vi "carwash_test.vi"() -> ()   [LabVIEW 2017]
panel:
  in  "Wash Selec.":enum16{"Initialize", "Deluxe", "Economy"}(ring)
  out "Vehicle Out of Position":bool
  out "Air Dry":bool
  out "Clear Water Rinse":bool
  out "Main High Press. Wash":bool
  out "Soap Application":bool
  out "Under body Wash":bool
  in  "?":bool
  in  "?":bool
  in  "?":bool
  in  "stop":bool
  # "Car Wash Indicators"
  # "Underbody wash\nposition \nSwitch"
  # "Main Wash \nPosition \nSwitch"
  # "Air Dry\nPosition\nSwitch"
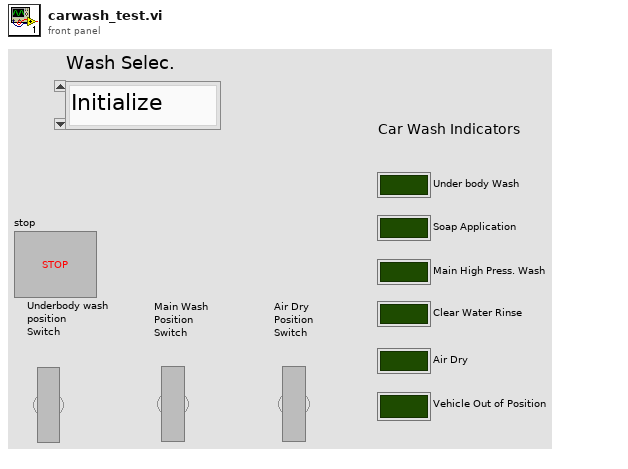
[diagram p1: front panel]
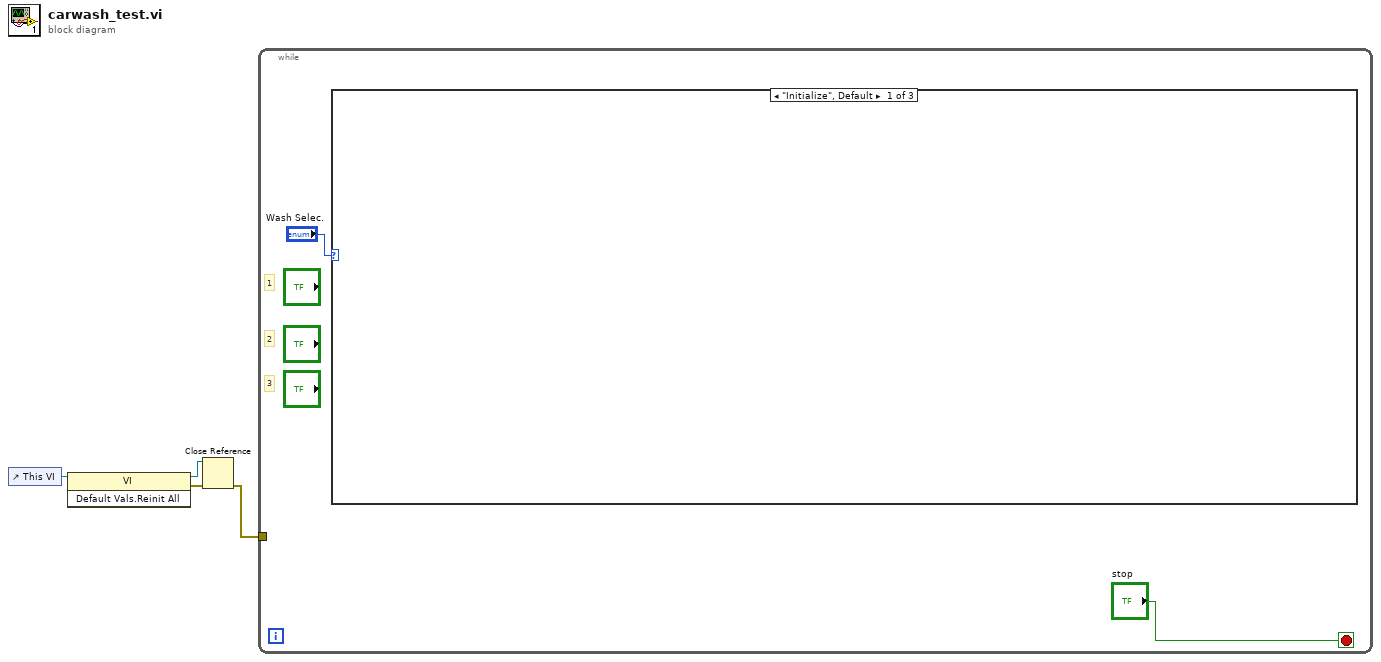
[diagram p0: block diagram]
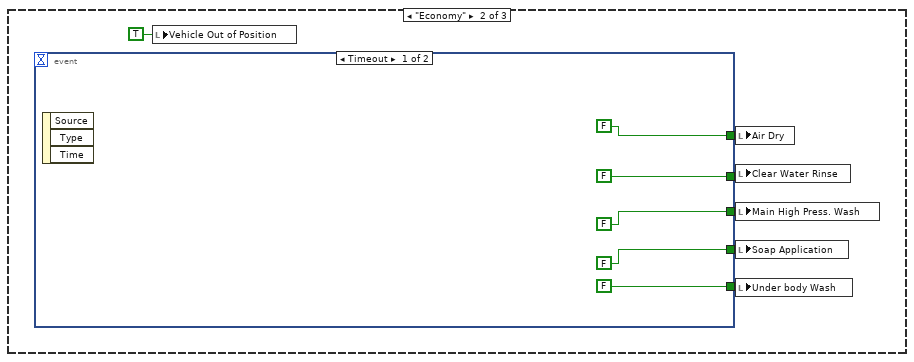
[diagram p2: hidden frame]
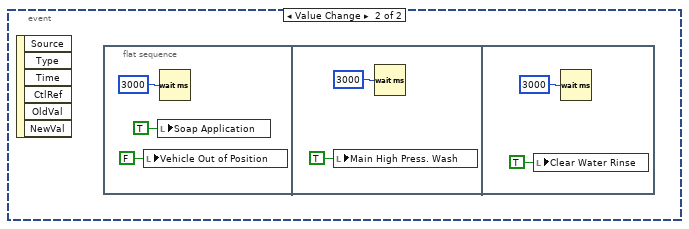
[diagram p3: hidden frame]
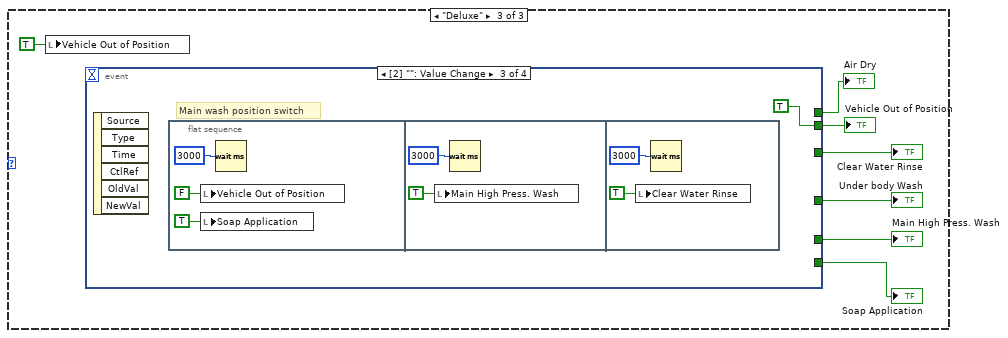
[diagram p4: hidden frame]
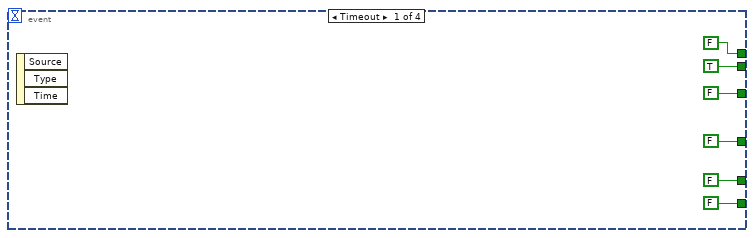
[diagram p5: hidden frame]
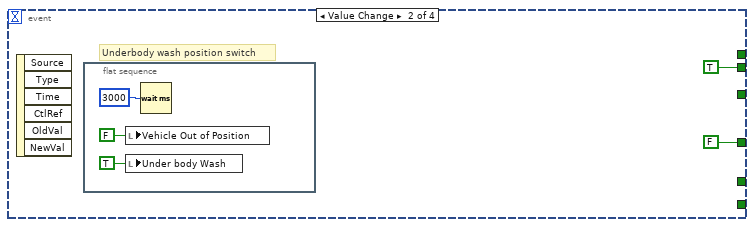
[diagram p6: hidden frame]
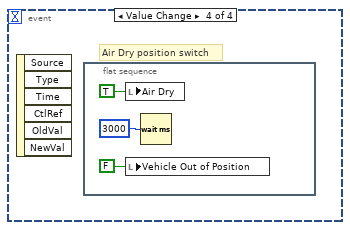
[diagram p7: hidden frame]
diagram:
  n1 = control-ref of="This VI"() -> (w3:refnum<vi>)
  n2 = invoke class="VI" method="Default Vals.Reinit All"(reference=w3) -> (reference out=w2:refnum<vi>, error out=w1:errorcluster)  [unwired: 2 in, 1 out]
  n3 = Close Reference(reference=w2, error in (no error)=w1) -> (error out=w4:errorcluster)
  n4 = while {
    tunnel: w4 -> [_]
    stop <- "stop" stop-if-true
    # "3"
    # "1"
    # "2"
    n5 = case shown="\"Initialize\", Default" "Wash Selec." {
      frame "Initialize", Default {
      }
      frame "Economy" {
        n6 = event shown="[0] Timeout" {
          selector: _ -> [_ _]
          dyn-events: _ -> [_ _]
          timeout: _ -> [_ _]
          tunnel: [FALSE _] -> w8
          tunnel: [FALSE _] -> w9
          tunnel: [FALSE _] -> w10
          tunnel: [FALSE _] -> w11
          tunnel: [FALSE _] -> w12
          event Timeout {
            n7 = event-data() -> ()  [unwired: 1 in, 3 out]
          }
          event Value Change {
            n8 = event-data() -> ()  [unwired: 1 in, 6 out]
            n9 = flat-sequence {
              frame #0 {
                n10 = local write "Vehicle Out of Position"(FALSE ("Vehicle Out of Position")) -> ()
                n11 = local write "Soap Application"(TRUE ("Soap Application")) -> ()
                n12 = Wait (ms)(milliseconds to wait=u32 3000) -> ()  [unwired: 1 out]
              }
              frame #1 {
                n13 = local write "Main High Press. Wash"(TRUE ("Main High Press. Wash")) -> ()
                n14 = Wait (ms)(milliseconds to wait=u32 3000) -> ()  [unwired: 1 out]
              }
              frame #2 {
                n15 = local write "Clear Water Rinse"(TRUE ("Clear Water Rinse")) -> ()
                n16 = Wait (ms)(milliseconds to wait=u32 3000) -> ()  [unwired: 1 out]
              }
            }
          }
        }
        n17 = local write "Vehicle Out of Position"(TRUE ("Vehicle Out of Position")) -> ()
        n18 = local write "Air Dry"(w8) -> ()
        n19 = local write "Clear Water Rinse"(w9) -> ()
        n20 = local write "Main High Press. Wash"(w10) -> ()
        n21 = local write "Soap Application"(w11) -> ()
        n22 = local write "Under body Wash"(w12) -> ()
      }
      frame "Deluxe" {
        n23 = local write "Vehicle Out of Position"(TRUE ("Vehicle Out of Position")) -> ()
        n24 = event shown="[2] \"\": Value Change" {
          selector: _ -> [_ _ _ _]
          dyn-events: _ -> [_ _ _ _]
          timeout: _ -> [_ _ _ _]
          tunnel: [FALSE FALSE _ _] -> w31
          tunnel: [FALSE _ _ _] -> w30
          tunnel: [FALSE _ _ _] -> w29
          tunnel: [FALSE _ _ _] -> w28
          tunnel: [FALSE _ _ _] -> w27
          tunnel: [TRUE TRUE TRUE _] -> w26
          event Timeout {
            n25 = event-data() -> ()  [unwired: 1 in, 3 out]
          }
          event Value Change {
            # "Underbody wash position switch"
            n26 = event-data() -> ()  [unwired: 1 in, 6 out]
            n27 = flat-sequence {
              frame #0 {
                n28 = local write "Vehicle Out of Position"(FALSE ("Vehicle Out of Position")) -> ()
                n29 = local write "Under body Wash"(TRUE ("Under body Wash")) -> ()
                n30 = Wait (ms)(milliseconds to wait=u32 3000) -> ()  [unwired: 1 out]
              }
            }
          }
          event Value Change {
            # "Main wash position switch"
            n31 = event-data() -> ()  [unwired: 1 in, 6 out]
            n32 = flat-sequence {
              frame #0 {
                n33 = local write "Vehicle Out of Position"(FALSE ("Vehicle Out of Position")) -> ()
                n34 = local write "Soap Application"(TRUE ("Boolean 2")) -> ()
                n35 = Wait (ms)(milliseconds to wait=u32 3000) -> ()  [unwired: 1 out]
              }
              frame #1 {
                n36 = local write "Main High Press. Wash"(TRUE ("Boolean 4")) -> ()
                n37 = Wait (ms)(milliseconds to wait=u32 3000) -> ()  [unwired: 1 out]
              }
              frame #2 {
                n38 = local write "Clear Water Rinse"(TRUE ("Boolean 4")) -> ()
                n39 = Wait (ms)(milliseconds to wait=u32 3000) -> ()  [unwired: 1 out]
              }
            }
          }
          event Value Change {
            # "Air Dry position switch"
            n40 = event-data() -> ()  [unwired: 1 in, 6 out]
            n41 = flat-sequence {
              frame #0 {
                n42 = local write "Air Dry"(TRUE ("Air Dry")) -> ()
                n43 = local write "Vehicle Out of Position"(FALSE ("Vehicle Out of Position")) -> ()
                n44 = Wait (ms)(milliseconds to wait=u32 3000) -> ()  [unwired: 1 out]
              }
            }
          }
        }
        "Under body Wash" <- w31
        "Soap Application" <- w30
        "Main High Press. Wash" <- w29
        "Clear Water Rinse" <- w28
        "Air Dry" <- w27
        "Vehicle Out of Position" <- w26
      }
    }
  }
